vi "Get Object by Ctl-Ref.vi"(8 "error in":errorcluster, 10 "Ctl Ref in":refnum<vi>, 11 "Button Manager in":refnum<class "Button Manager.lvclass">) -> (0 "error out":errorcluster, 2 "Button Object":T1, 3 "Button Manager out":refnum<class "Button Manager.lvclass">, 5 "Sub-Ctl Ref":refnum<vi>, 7 "Top-Ctl Ref":refnum<vi>)   [LabVIEW 2022 SP3, in "Navigation.lvlib" / "Button Manager.lvclass"]
doc: "____\nHAMPEL SOFTWARE ENGINEERING v2.6.0 (2023-12-19 10:54)"
uses:
  Button Manager.lvclass
  Top Control.ctl
  Sub Control.ctl
  Button Manager.lvclass/Button Manager.ctl
  Button Def.ctl
  <vilib>/Utility/error.llb/Error Cluster From Error Code.vi
  <vilib>/ErrorRing/Error Ring.xnode
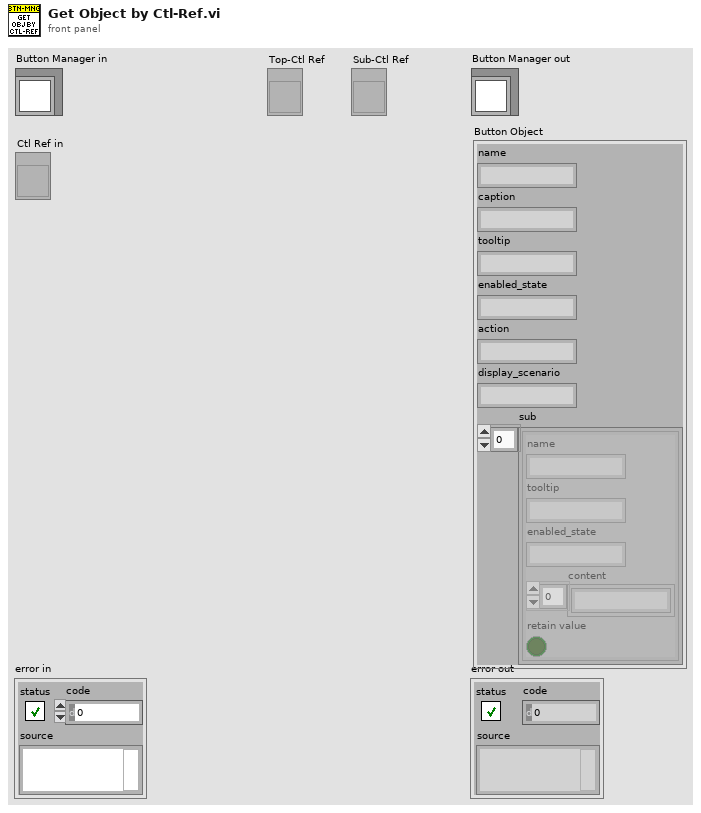
[diagram p1: front panel]
types:
  T1 = typedef "Navigation.lvlib/Button Manager.lvclass/Top Control.ctl" = cluster{"name":string, "caption":string, "tooltip":string, "enabled_state":string, "action":string, "display_scenario":string, "sub":T2[]}
  T2 = typedef "Navigation.lvlib/Button Manager.lvclass/Sub Control.ctl" = cluster{"name":string, "tooltip":string, "enabled_state":string, "content":string[], "retain value":bool}
  T3 = typedef "Navigation.lvlib/Button Manager.lvclass/Button Def.ctl" = cluster{"Top-Ctl Ref":refnum<vi>, "Sub-Ctl Ref":refnum<vi>, "Button Object":T1}
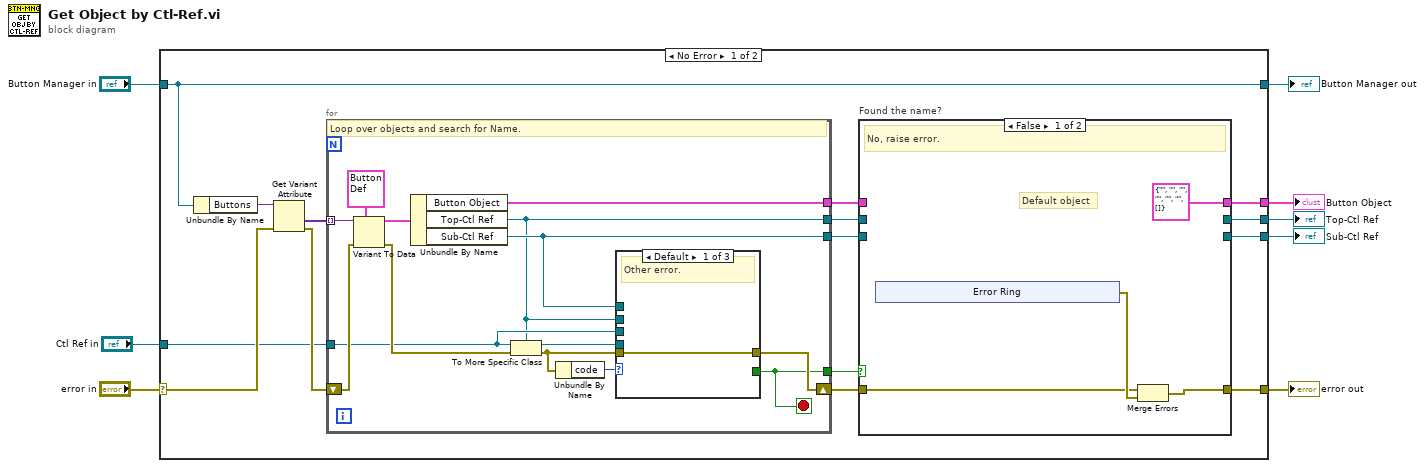
[diagram p0: block diagram]
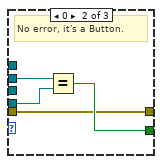
[diagram p3: hidden frame]
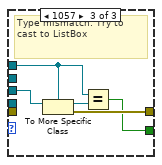
[diagram p4: hidden frame]
diagram:
  n1 = case shown="No Error" "error in" {
    selector: "error in" -> [w20 w63]
    tunnel: [w15 w63] -> w7
    tunnel: [w22 w62] -> w5
    tunnel: "Button Manager in" -> [w22 w62]
    tunnel: "Ctl Ref in" -> [w17 _]
    tunnel: [w13 _] -> w4
    tunnel: [w10 _] -> w2
    tunnel: [w9 _] -> w1
    frame No Error {
      n2 = Unbundle By Name(w22) -> ("Buttons"=w21:variant)
      n3 = Get Variant Attribute(Variant=w21, error in=w20) -> (values=w19:variant[], error out=w18:errorcluster)  [unwired: 2 in, 2 out]
      n4 = for {
        tunnel: w19 -> [w50] mode=indexing
        tunnel: w17 -> [w42]
        tunnel: [w39] -> w16
        shift-right: [w40] -> w23
        shift-left: w18 -> [w49]
        tunnel: [w46] -> w14
        tunnel: [w38] -> w11
        tunnel: [w37] -> w12
        stop <- w39 stop-if-true
        # "Loop over objects and search for Name."
        n5 = Variant To Data(error in=w49, type=T3 {"Top-Ctl Ref"=refnum, "Sub-Ctl Ref"=refnum, "Button Object"={"name"="", "caption"="", "tooltip"="", "enabled_state"="", "action"="", "display_scenario"="", "sub"=[]}} ("Button Def"), Variant=w50) -> (data=w47:T3, error out=w45:errorcluster)
        n6 = Unbundle By Name(w47) -> ("Button Object"=w46:T1, "Top-Ctl Ref"=w37:refnum<vi>, "Sub-Ctl Ref"=w38:refnum<vi>)
        n7 = To More Specific Class(target class=w37, reference=w42, error in=w45) -> (specific class reference=w43:refnum<vi>, error out=w41:errorcluster)
        n8 = Unbundle By Name(w41) -> ("code"=w44:i32)
        n9 = case shown="Default" w44 {
          tunnel: w43 -> [_ w56 _]
          tunnel: w42 -> [_ _ w61]
          tunnel: w41 -> [w52 w53 _]
          tunnel: [w52 w53 w59] -> w40
          tunnel: [FALSE w54 w58] -> w39
          tunnel: w38 -> [_ _ w57]
          tunnel: w37 -> [_ w55 _]
          frame Default {
            # "Other error."
          }
          frame 0 {
            # "No error, it's a Button."
            n10 = Equal?(x=w55, y=w56) -> (x = y?=w54:bool)
          }
          frame 1057 {
            # "Type mismatch. Try to cast to ListBox"
            n11 = To More Specific Class(target class=w57, reference=w61) -> (specific class reference=w60:refnum<vi>, error out=w59:errorcluster)  [unwired: 1 in]
            n12 = Equal?(x=w57, y=w60) -> (x = y?=w58:bool)
          }
        }
      }
      n13 = case "Found the name?" shown="False" w16 {
        tunnel: w23 -> [w26 w33]
        tunnel: [w25 w33] -> w15
        tunnel: w14 -> [_ w34]
        tunnel: [T1 {"name"="", "caption"="", "tooltip"="", "enabled_state"="", "action"="", "display_scenario"="", "sub"=[]} ("Button Object") w34] -> w13
        tunnel: [_ w36] -> w10
        tunnel: w12 -> [_ w36]
        tunnel: [_ w35] -> w9
        tunnel: w11 -> [_ w35]
        frame False {
          # "Default object"
          # "No, raise error."
          n14 = xnode "Error Ring"() -> ("error out"=w27:errorcluster)
          n15 = Merge Errors(w26, w27) -> (w25:errorcluster)
        }
        frame True {
          # "Yes"
        }
      }
    }
    frame Error {
    }
  }
  "error out" <- w7
  "Button Manager out" <- w5
  "Button Object" <- w4
  "Top-Ctl Ref" <- w2
  "Sub-Ctl Ref" <- w1
